vi "List Available Measurements.vi"(8 "error in (no error)":errorcluster, 10 "enumerate services request":T1, 11 "multicolumnListbox ref in":refnum<vi>) -> (0 "error out":errorcluster, 1 "warning":string, 2 "available measurement details":T2, 3 "multicolumnListbox ref":refnum<vi>)   [LabVIEW 2021, in "MeasurementClient Editor.lvlib"]
uses:
  MeasurementClient Editor.lvlib
  <vilib>/gRPC/Generated APIs/ni/measurementlink/discovery/v1/RPC Messages/ni_measurementlink_discovery_v1_EnumerateServicesResponse.ctl
  <vilib>/gRPC/Generated APIs/ni/measurementlink/discovery/v1/RPC Messages/ni_measurementlink_discovery_v1_ServiceDescriptor.ctl
  <vilib>/gRPC/Generated APIs/ni/measurementlink/discovery/v1/RPC Messages/ni_measurementlink_discovery_v1_ServiceDescriptor_AnnotationsEntry.ctl
  <vilib>/gRPC/Generated APIs/ni/measurementlink/discovery/v1/RPC Messages/ni_measurementlink_discovery_v1_EnumerateServicesRequest.ctl
  <vilib>/Utility/miscctls.llb/LVRowAndColumnTypeDef.ctl
  <vilib>/Plug-In SDKs/Clients/Discovery V1/NI Discovery V1 Client.lvlib
  <vilib>/gRPC/Generated APIs/ni/measurementlink/discovery/v1/ni.measurementlink.discovery.v1.api.lvlib
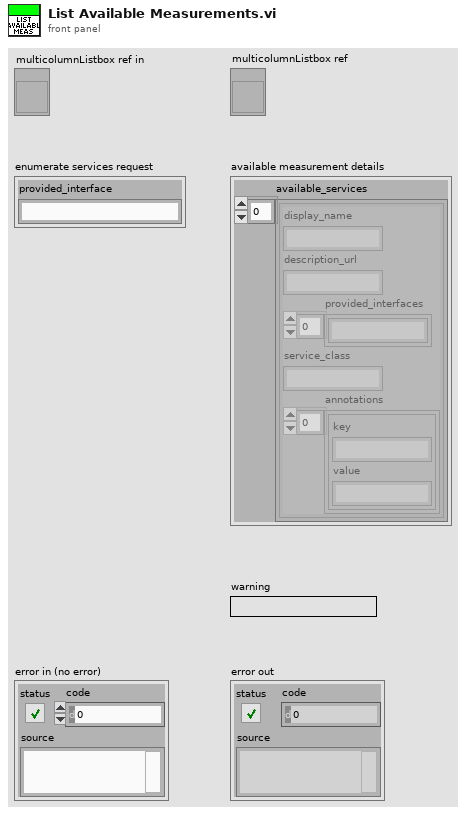
[diagram p1: front panel]
types:
  T1 = typedef "ni.measurementlink.discovery.v1.api.lvlib/ni_measurementlink_discovery_v1_EnumerateServicesRequest.ctl" = cluster{"provided_interface":string}
  T2 = typedef "ni.measurementlink.discovery.v1.api.lvlib/ni_measurementlink_discovery_v1_EnumerateServicesResponse.ctl" = cluster{"available_services":T3[]}
  T3 = typedef "ni.measurementlink.discovery.v1.api.lvlib/ni_measurementlink_discovery_v1_ServiceDescriptor.ctl" = cluster{"display_name":string, "description_url":string, "provided_interfaces":string[], "service_class":string, "annotations":T4[]}
  T4 = typedef "ni.measurementlink.discovery.v1.api.lvlib/ni_measurementlink_discovery_v1_ServiceDescriptor_AnnotationsEntry.ctl" = cluster{"key":string, "value":string}
  T5 = typedef "LVRowAndColumnTypeDef.ctl" = cluster{"Row":i32, "Column":i32}
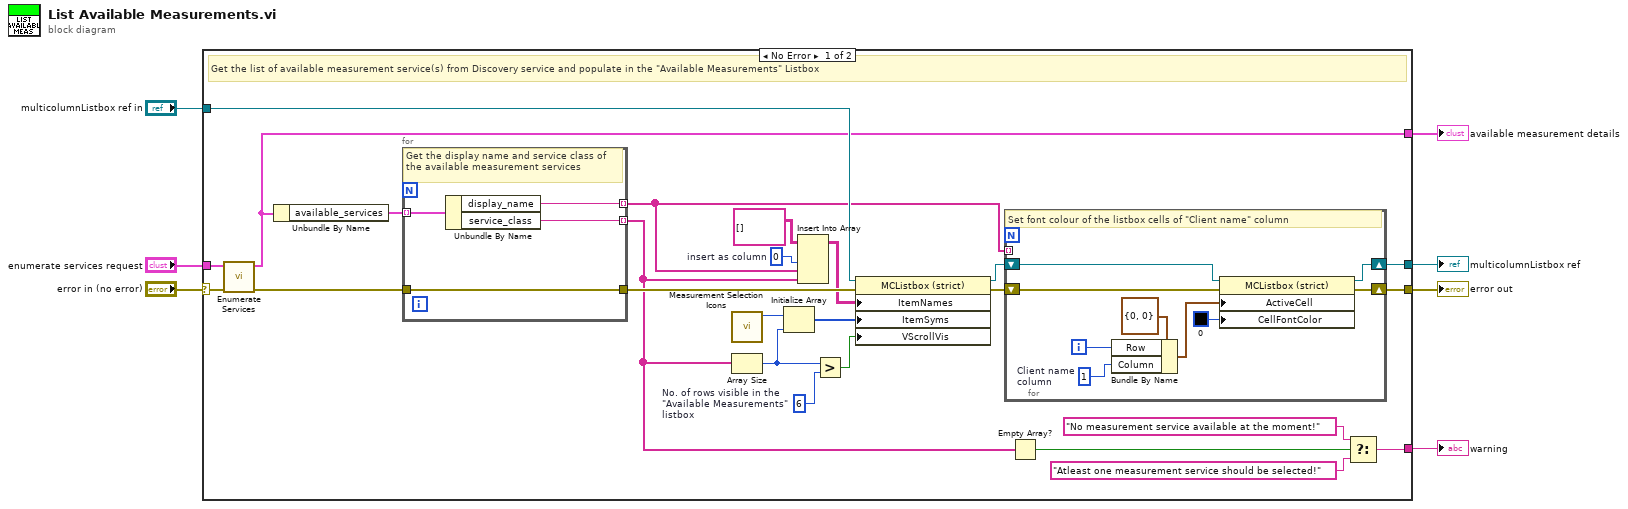
[diagram p0: block diagram]
diagram:
  n1 = case shown="No Error" "error in (no error)" {
    selector: "error in (no error)" -> [w27 w46]
    tunnel: [w22 w46] -> w7
    tunnel: "multicolumnListbox ref in" -> [w31 w47]
    tunnel: [w19 w47] -> w5
    tunnel: [w30 _] -> w4
    tunnel: [w26 _] -> w2
    tunnel: "enumerate services request" -> [w25 _]
    frame No Error {
      w14 = 0  # insert as column
      w28 = 6  # No. of rows visible in the "Available Measurements" listbox
      # "Get the list of available measurement service(s) from Discovery service and populate in the \"Available Measurements\" Listbox"
      n2 = call <vilib>:"Enumerate Services.vi"("error in"=w27, "request data"=w25) -> ("error out"=w20:errorcluster, "response data"=w26:T2)  [unwired: 7 in]
      n3 = Unbundle By Name(w26) -> ("available_services"=w15:T3[])
      n4 = for {
        tunnel: w15 -> [w36] mode=indexing
        tunnel: [w35] -> w16 mode=indexing
        tunnel: [w33] -> w32
        tunnel: w20 -> [w33]
        tunnel: [w34] -> w9 mode=indexing
        # "Get the display name and service class of the available measurement services"
        n5 = Unbundle By Name(w36) -> ("display_name"=w34:string, "service_class"=w35:string)
      }
      n6 = call "Measurement Selection Icons.vi"() -> ("Unchecked"=w12:i32)  [unwired: 10 in, 1 out]
      n7 = Array Size(array=w16) -> (size(s)=w11:i32)
      n8 = Initialize Array(w12, w11) -> (w10:i32[])
      n9 = Insert Into Array(array=string[][] [], index (col)=w14, new element #1=w9, new element #2=w16) -> (w17:string[][])  [unwired: 1 in]
      n10 = Greater?(x=w11, y=w28) -> (0:w13:bool)
      n11 = property class="MCListbox (strict)"(reference=w31, error in=w32, "ItemNames"=w17, "ItemSyms"=w10, "VScrollVis"=w13) -> (reference out=w21:refnum<vi>, error out=w23:errorcluster)
      n12 = for {
        shift-right: [w44] -> w22
        shift-left: w23 -> [w45]
        tunnel: w9 -> [_] mode=indexing
        shift-right: [w38] -> w19
        shift-left: w21 -> [w43]
        i -> [w40]
        w37 = 1  # Client name column
        # "Set font colour of the listbox cells of \"Client name\" column"
        n13 = Bundle By Name(cluster=T5 {"Row"=0, "Column"=0} ("Active Cell:Active Cell"), "Row"=w40, "Column"=w37) -> (w41:T5)
        n14 = property class="MCListbox (strict)"(reference=w43, error in=w45, "ActiveCell"=w41, "CellFontColor"=u32 0 ("Active Cell:Cell Font:Color")) -> (reference out=w38:refnum<vi>, error out=w44:errorcluster)
      }
      n15 = Empty Array?(array=w16) -> (empty?=w8:bool)
      n16 = Select(t="No measurement service available at the moment!", s=w8, f="Atleast one measurement service should be selected!") -> (s? t:f=w30:string)
    }
    frame Error {
      # "Pass"
    }
  }
  "error out" <- w7
  "multicolumnListbox ref" <- w5
  "warning" <- w4
  "available measurement details" <- w2
